vi "tt20panel_DO_chart_counts.vi"(8 "error in (no error)":errorcluster, 10 "stop_counts":refnum<queue>, 11 "tt20panel in":refnum<class "tt20panel.lvclass">) -> (0 "error out":errorcluster, 3 "tt20panel out":refnum<class "tt20panel.lvclass">)   [LabVIEW 2015, in "tt20panel.lvclass"]
uses:
  tt20panel.lvclass
  tt20_class/tt20.lvclass
  UI/panel_class/panel.lvclass
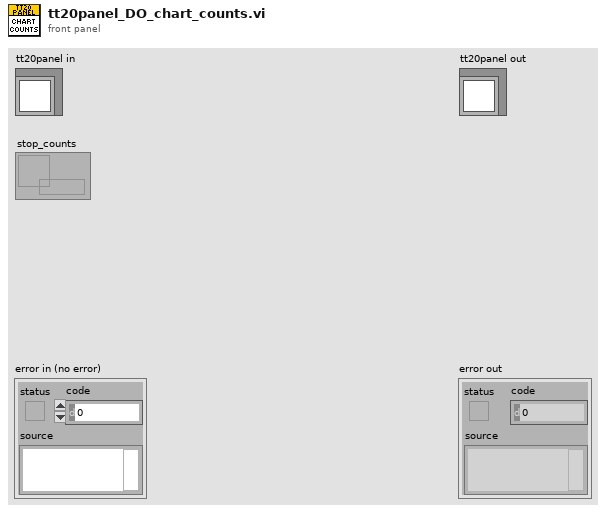
[diagram p1: front panel]
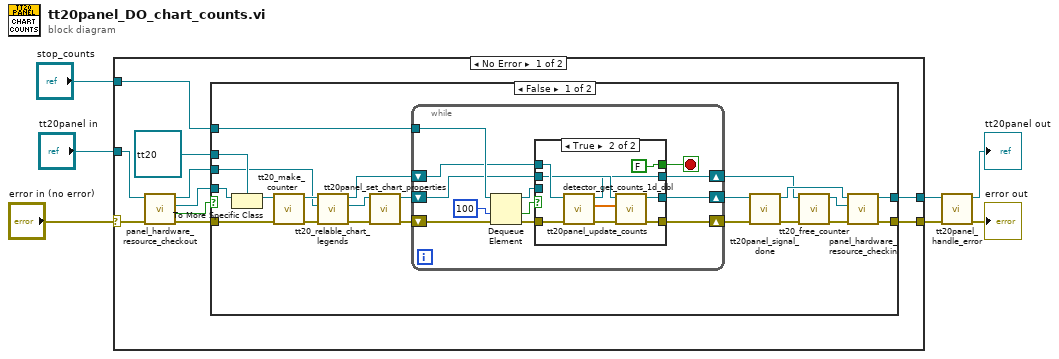
[diagram p0: block diagram]
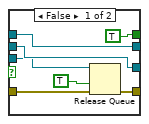
[diagram p2: hidden frame]
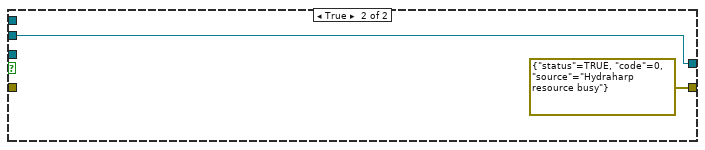
[diagram p3: hidden frame]
diagram:
  n1 = case shown="No Error" "error in (no error)" {
    selector: "error in (no error)" -> [w16 w71]
    tunnel: [w13 w71] -> w5
    tunnel: [w10 w70] -> w1
    tunnel: "tt20panel in" -> [w17 w70]
    tunnel: "stop_counts" -> [w8 _]
    frame No Error {
      n2 = call "panel_hardware_resource_checkout.vi"("error in (no error)"=w16, "panel in"=w17) -> ("error out"=w14:errorcluster, "timed out?"=w15:bool, "hardware.lvclass"=w11:refnum<class "hardware.lvclass">, "panel out"=w12:refnum<class "tt20panel.lvclass">)  [unwired: 6 in]
      n3 = case shown="False" w15 {
        tunnel: w14 -> [w29 _]
        tunnel: [w37 errorcluster {"status"=TRUE, "code"=0, "source"="Hydraharp resource busy"} ("error out")] -> w13
        tunnel: w12 -> [w21 w68]
        tunnel: w11 -> [w38 _]
        tunnel: refnum<class "tt20.lvclass"> refnum ("tt20.lvclass") -> [w39 _]
        tunnel: [w36 w68] -> w10
        tunnel: w8 -> [w35 _]
        frame False {
          n4 = To More Specific Class(target class=w39, reference=w38) -> (specific class reference=w28:refnum<class "tt20.lvclass">)  [unwired: 1 in, 1 out]
          n5 = call "tt20_make_counter.vi"("error in (no error)"=w29, "tt20 in"=w28) -> ("error out"=w23:errorcluster, "tt20 out"=w22:refnum<class "tt20.lvclass">)  [unwired: 8 in]
          n6 = call "tt20_relable_chart_legends.vi"("error in (no error)"=w23, "panel in"=w21, "tt20 in"=w22) -> ("error out"=w18:errorcluster, "panel out"=w20:refnum<class "tt20panel.lvclass">, "tt20 out"=w19:refnum<class "tt20.lvclass">)  [unwired: 6 in]
          n7 = call "tt20panel_set_chart_properties.vi"("error in (no error)"=w18, "panel.lvclass"=w20) -> ("error in (no error) 2"=w34:errorcluster, "panel out"=w33:refnum<class "tt20panel.lvclass">)  [unwired: 8 in]
          n8 = while {
            tunnel: w35 -> [w51]
            shift-right: [w43] -> w32
            shift-left: w34 -> [w49]
            shift-right: [w44] -> w25
            shift-left: w19 -> [w46]
            shift-right: [w42] -> w31
            shift-left: w33 -> [w45]
            stop <- w41 stop-if-true
            n9 = Dequeue Element(queue=w51, timeout in ms (-1)=100, error in (no error)=w49) -> (queue out=w40:refnum<queue>, timed out?=w48:bool, error out=w47:errorcluster)  [unwired: 1 out]
            n10 = case shown="True" w48 {
              tunnel: w47 -> [w54 w67]
              tunnel: w46 -> [w57 w66]
              tunnel: w45 -> [w56 w65]
              tunnel: [w57 w62] -> w44
              tunnel: [w53 w61] -> w43
              tunnel: [w56 w60] -> w42
              tunnel: [TRUE FALSE] -> w41
              tunnel: w40 -> [w55 _]
              frame False {
                n11 = Release Queue(queue=w55, force destroy? (F)=TRUE, error in (no error)=w54) -> (error out=w53:errorcluster)  [unwired: 2 out]
              }
              frame True {
                n12 = call-dynamic "detector_get_counts_1d_dbl.vi"("error in (no error)"=w67, "tt20 in"=w66) -> ("error out"=w64:errorcluster, "counts"=w63:dbl[], "tt20 out"=w62:refnum<class "tt20.lvclass">)  [unwired: 7 in]
                n13 = call "tt20panel_update_counts.vi"("error in (no error)"=w64, "Counts"=w63, "tt20panel in"=w65) -> ("error out"=w61:errorcluster, "tt20panel out"=w60:refnum<class "tt20panel.lvclass">)  [unwired: 7 in]
              }
            }
          }
          n14 = call "tt20panel_signal_done.vi"("error in (no error)"=w32, "tt20panel in"=w31) -> ("error out"=w27:errorcluster, "tt20panel out"=w30:refnum<class "tt20panel.lvclass">)  [unwired: 8 in]
          n15 = call "tt20_free_counter.vi"("error in (no error)"=w27, "tt20 in"=w25) -> ("error out"=w26:errorcluster, "tt20 out"=w24:refnum<class "tt20.lvclass">)  [unwired: 8 in]
          n16 = call "panel_hardware_resource_checkin.vi"("error in (no error)"=w26, "hardware.lvclass"=w24, "panel in"=w30) -> ("error out"=w37:errorcluster, "panel out"=w36:refnum<class "tt20panel.lvclass">)  [unwired: 7 in]
        }
        frame True {
        }
      }
    }
    frame Error {
    }
  }
  n17 = call "tt20panel_handle_error.vi"("error in (no error)"=w5, "tt20panel in"=w1) -> ("error out"=→"error out":errorcluster, "tt20panel out"=→"tt20panel out":refnum<class "tt20panel.lvclass">)  [unwired: 8 in]
